vi "Get VIs in Project.vi"(7 "error in":errorcluster, 10 "Project in":refnum<vi>) -> (0 "error out":errorcluster, 2 "Results":T1, 3 "Project out":refnum<vi>)   [LabVIEW 2020]
uses:
  <vilib>/SourceOnly/NI_SourceOnly_CollectionOfVIsAndLibraries.ctl
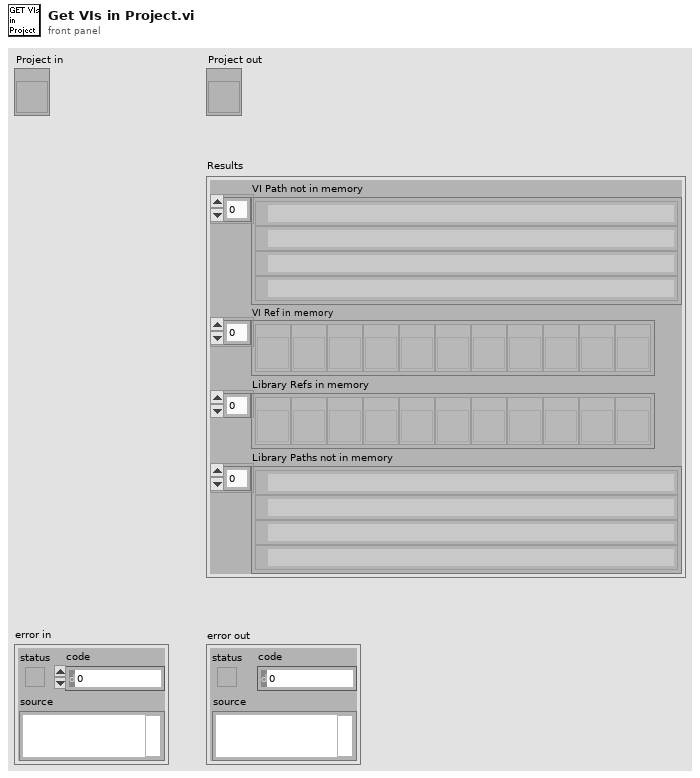
[diagram p1: front panel]
types:
  T1 = typedef "NI_SourceOnly_CollectionOfVIsAndLibraries.ctl" = cluster{"VI Path not in memory":path[], "VI Ref in memory":refnum<vi>[], "Library Refs in memory":refnum<vi>[], "Library Paths not in memory":path[]}
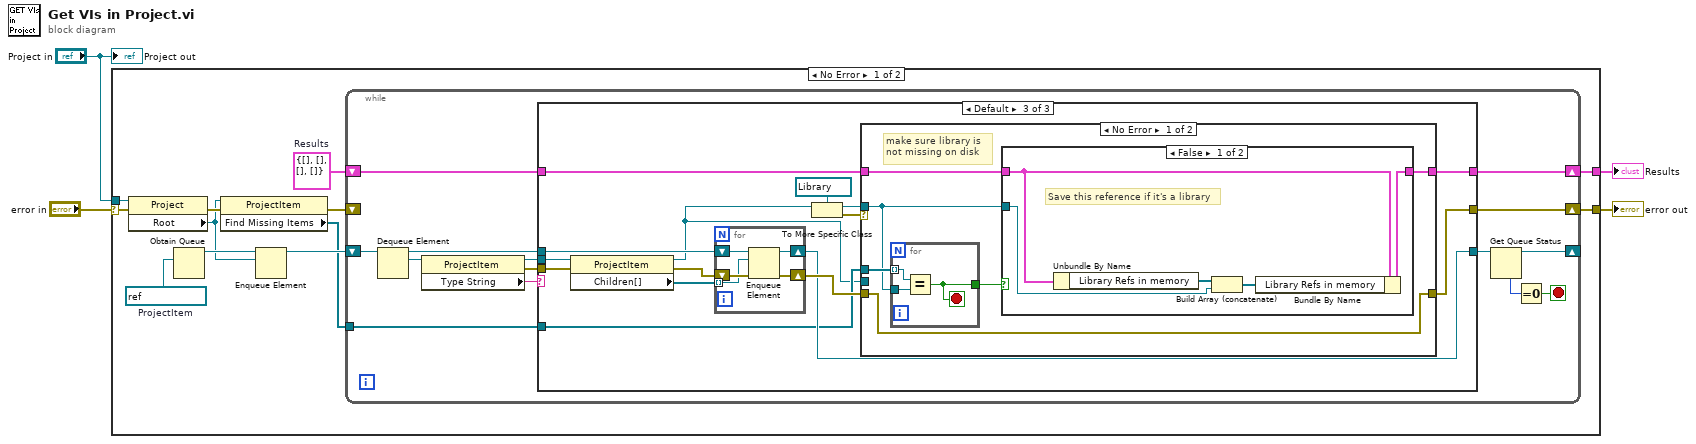
[diagram p0: block diagram]
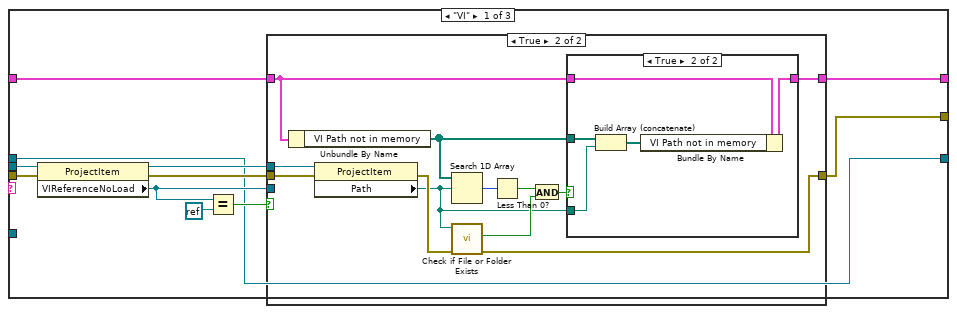
[diagram p2: hidden frame]
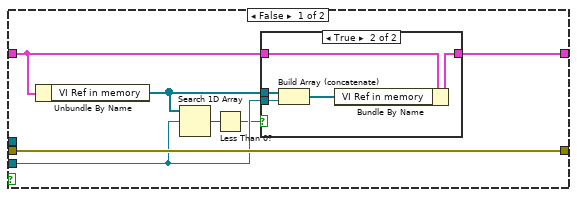
[diagram p3: hidden frame]
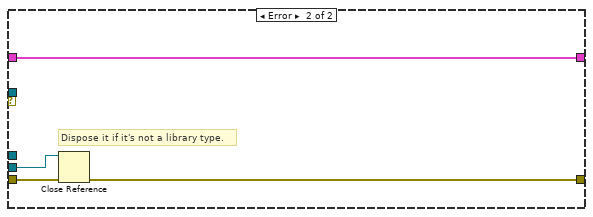
[diagram p8: hidden frame]
diagram:
  n1 = case shown="No Error" "error in" {
    selector: "error in" -> [w13 w115]
    tunnel: "Project in" -> [w12 _]
    tunnel: [w16 w115] -> w3
    tunnel: [w10 _] -> w1
    frame No Error {
      w9 = refnum<vi> refnum  # ProjectItem
      w11 = T1 {"VI Path not in memory"=[], "VI Ref in memory"=[], "Library Refs in memory"=[], "Library Paths not in memory"=[]}  # Results
      n2 = property class="Project"(reference=w12, error in=w13) -> (error out=w15:errorcluster, "Root"=w6:refnum<vi>)  [unwired: 1 out]
      n3 = Obtain Queue(element data type=w9) -> (queue out=w8:refnum<queue>)  [unwired: 4 in, 2 out]
      n4 = property class="ProjectItem"(reference=w6, error in=w15) -> (error out=w14:errorcluster, "Find Missing Items"=w5:refnum<vi>[])  [unwired: 1 out]
      n5 = Enqueue Element(queue=w8, element=w6) -> (queue out=w7:refnum<queue>)  [unwired: 2 in, 2 out]
      n6 = while {
        shift-right: [w18] -> _
        shift-left: w7 -> [w23]
        shift-right: [w30] -> w16
        shift-left: w14 -> [_]
        shift-right: [w26] -> w10
        shift-left: w11 -> [w27]
        tunnel: w5 -> [w17]
        stop <- w28 stop-if-true
        n7 = Dequeue Element(queue=w23) -> (queue out=w20:refnum<queue>, element=w22:refnum<vi>)  [unwired: 2 in, 2 out]
        n8 = property class="ProjectItem"(reference=w22) -> (reference out=w24:refnum<vi>, error out=w29:errorcluster, "Type String"=w21:string)  [unwired: 1 in]
        n9 = case shown="Default" w21 {
          tunnel: w24 -> [w34 _ w78]
          tunnel: w29 -> [w40 w75 w88]
          tunnel: [w39 w75 w86] -> w30
          tunnel: w27 -> [w33 w74 w83]
          tunnel: [w32 w74 w82] -> w26
          tunnel: w20 -> [w31 w73 w80]
          tunnel: [w31 w73 w79] -> w19
          tunnel: w17 -> [_ _ w77]
          frame "VI" {
            n10 = property class="ProjectItem"(reference=w34, error in=w40) -> (reference out=w36:refnum<vi>, error out=w41:errorcluster, "VIReferenceNoLoad"=w35:refnum<vi>)
            n11 = Equal?(x=w35, y=refnum<k0> refnum) -> (x = y?=w37:bool)
            n12 = case shown="True" w37 {
              tunnel: w36 -> [_ w63]
              tunnel: w41 -> [w48 w66]
              tunnel: [w48 w64] -> w39
              tunnel: w35 -> [w47 _]
              tunnel: w33 -> [w43 w56]
              tunnel: [w42 w57] -> w32
              frame False {
                n13 = Unbundle By Name(w43) -> ("VI Ref in memory"=w44:refnum<vi>[])
                n14 = Search 1D Array(1D array=w44, element=w47) -> (index of element=w46:i32)  [unwired: 1 out]
                n15 = Less Than 0?(x=w46) -> (x < 0?=w45:bool)
                n16 = case shown="True" w45 {
                  tunnel: w47 -> [_ w54]
                  tunnel: w44 -> [_ w53]
                  tunnel: w43 -> [w49 w52]
                  tunnel: [w49 w50] -> w42
                  frame False {
                  }
                  frame True {
                    n17 = Build Array (concatenate)(w53, w54) -> (w51:refnum<vi>[])
                    n18 = Bundle By Name(cluster=w52, "VI Ref in memory"=w51) -> (w50:T1)
                  }
                }
              }
              frame True {
                n19 = Unbundle By Name(w56) -> ("VI Path not in memory"=w55:path[])
                n20 = property class="ProjectItem"(reference=w63, error in=w66) -> (error out=w65:errorcluster, "Path"=w58:path)  [unwired: 1 out]
                n21 = Search 1D Array(1D array=w55, element=w58) -> (index of element=w62:i32)  [unwired: 1 out]
                n22 = call <vilib>:"Check if File or Folder Exists.vi"("error in (no error)"=w65, "path"=w58) -> ("error out"=w64:errorcluster, "file or folder exists?"=w61:bool)  [unwired: 8 out]
                n23 = Less Than 0?(x=w62) -> (x < 0?=w60:bool)
                n24 = And(x=w60, y=w61) -> (x .and. y?=w59:bool)
                n25 = case shown="True" w59 {
                  tunnel: w56 -> [w67 w72]
                  tunnel: w58 -> [_ w71]
                  tunnel: [w67 w69] -> w57
                  tunnel: w55 -> [_ w68]
                  frame False {
                  }
                  frame True {
                    n26 = Build Array (concatenate)(w68, w71) -> (w70:path[])
                    n27 = Bundle By Name(cluster=w72, "VI Path not in memory"=w70) -> (w69:T1)
                  }
                }
              }
            }
          }
          frame "Dependencies" {
            # "Intentionally avoid queue-ing up items under the 'dependencies' folder."
          }
          frame Default {
            n28 = property class="ProjectItem"(reference=w78, error in=w88) -> (reference out=w76:refnum<vi>, error out=w89:errorcluster, "Children[]"=w81:refnum<vi>[])
            n29 = for {
              tunnel: w81 -> [w92] mode=indexing
              shift-right: [w94] -> w87
              shift-left: w89 -> [w95]
              shift-right: [w91] -> w79
              shift-left: w80 -> [w93]
              n30 = Enqueue Element(queue=w93, element=w92, error in (no error)=w95) -> (queue out=w91:refnum<queue>, error out=w94:errorcluster)  [unwired: 1 in, 1 out]
            }
            n31 = To More Specific Class(target class=refnum<vi> refnum ("reference out"), reference=w76) -> (specific class reference=w84:refnum<vi>, error out=w90:errorcluster)  [unwired: 1 in]
            n32 = case shown="No Error" w90 {
              tunnel: w84 -> [w96 _]
              tunnel: [w100 w112] -> w82
              tunnel: w83 -> [w99 w112]
              tunnel: w87 -> [w101 w114]
              tunnel: [w101 w113] -> w86
              tunnel: w76 -> [_ w111]
              tunnel: w77 -> [w97 _]
              frame No Error {
                # "make sure library is not missing on disk"
                n33 = for {
                  tunnel: w97 -> [w110] mode=indexing
                  tunnel: w96 -> [w109]
                  tunnel: [w108] -> w98
                  stop <- w108 stop-if-true
                  n34 = Equal?(x=w110, y=w109) -> (x = y?=w108:bool)
                }
                n35 = case shown="False" w98 {
                  tunnel: [w105 w107] -> w100
                  tunnel: w99 -> [w104 w107]
                  tunnel: w96 -> [w102 _]
                  frame False {
                    # "Save this reference if it's a library"
                    n36 = Unbundle By Name(w104) -> ("Library Refs in memory"=w103:refnum<vi>[])
                    n37 = Build Array (concatenate)(w103, w102) -> (w106:refnum<vi>[])
                    n38 = Bundle By Name(cluster=w104, "Library Refs in memory"=w106) -> (w105:T1)
                  }
                  frame True {
                  }
                }
              }
              frame Error {
                # "Dispose it if it's not a library type."
                n39 = Close Reference(reference=w111, error in (no error)=w114) -> (error out=w113:errorcluster)
              }
            }
          }
        }
        n40 = Get Queue Status(queue=w19) -> (queue out=w18:refnum<queue>, # elements in queue=w25:i32)  [unwired: 2 in, 6 out]
        n41 = Equal To 0?(x=w25) -> (x = 0?=w28:bool)
      }
    }
    frame Error {
    }
  }
  "error out" <- w3
  "Results" <- w1
  "Project out" <- "Project in"
